vi "Calculate Index Array.vi"(8 "error in (no error)":errorcluster, 10 "3D Surface Datatype.lvclass in":refnum<class "3D Surface Datatype.lvclass">, 11 "Plot Representation In":T1) -> (0 "error out":errorcluster, 2 "3D Surface Datatype.lvclass out":refnum<class "3D Surface Datatype.lvclass">, 3 "Plot Representation Out":T1)   [LabVIEW 2020, in "3D Surface Datatype.lvclass"]
uses:
  <vilib>/Math Plots/3D Math Plots/3D Surface/3D Surface Datatype/3D Surface Datatype.lvclass
  <vilib>/Math Plots/3D Math Plots/3D Plot/3D Plot/Typedef/Plot Representation.ctl
  <vilib>/Math Plots/3D Math Plots/3D Plot/3D Plot/Typedef/Range Clusters.ctl
  <vilib>/Math Plots/3D Math Plots/3D Plot/3D Plot/Typedef/Mesh Data.ctl
  <vilib>/Math Plots/3D Math Plots/3D Plot/3D Plot/3D Plot.lvclass
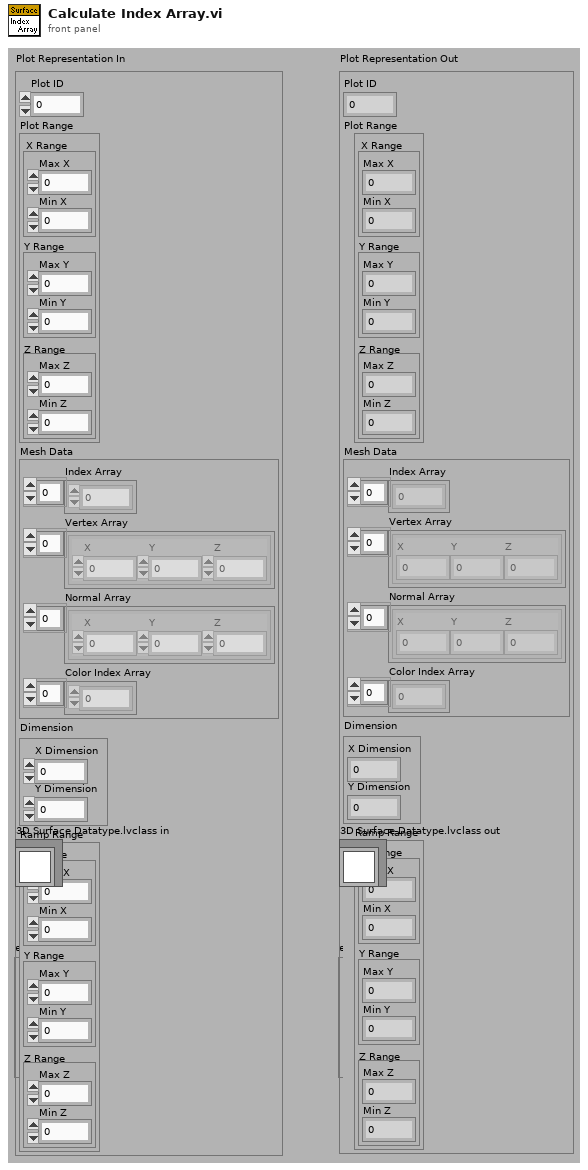
[diagram p1: front panel]
types:
  T1 = typedef "3D Plot.lvclass/Plot Representation.ctl" = cluster{"Plot ID":i32, "Plot Range":T2, "Mesh Data":T3, "Dimension":cluster{"X Dimension":i32, "Y Dimension":i32}, "Ramp Range":T2}
  T2 = typedef "3D Plot.lvclass/Range Clusters.ctl" = cluster{"X Range":cluster{"Max X":sgl, "Min X":sgl}, "Y Range":cluster{"Max Y":sgl, "Min Y":sgl}, "Z Range":cluster{"Max Z":sgl, "Min Z":sgl}}
  T3 = typedef "3D Plot.lvclass/Mesh Data.ctl" = cluster{"Index Array":u32[], "Vertex Array":cluster{"X":sgl, "Y":sgl, "Z":sgl}[], "Normal Array":cluster{"X":sgl, "Y":sgl, "Z":sgl}[], "Color Index Array":i32[]}
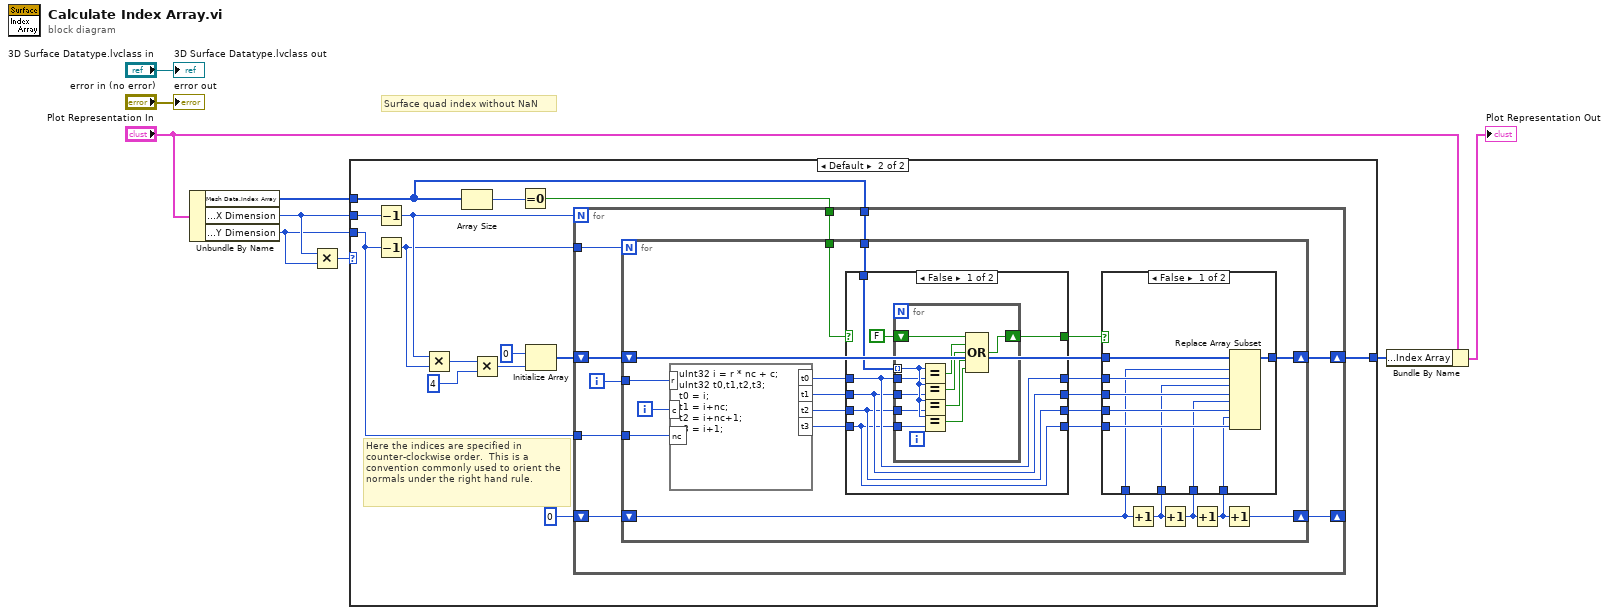
[diagram p0: block diagram]
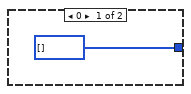
[diagram p2: hidden frame]
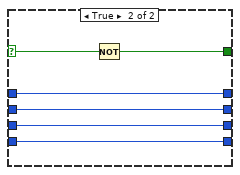
[diagram p3: hidden frame]
diagram:
  # "Surface quad index without NaN"
  n1 = Unbundle By Name("Plot Representation In") -> ("Mesh Data.Index Array"=w1:u32[], "Dimension.X Dimension"=w4:i32, "Dimension.Y Dimension"=w3:i32)
  n2 = Multiply(x=w4, y=w3) -> (x*y=w2:i32)
  n3 = case shown="Default" w2 {
    tunnel: w4 -> [_ w24]
    tunnel: w3 -> [_ w23]
    tunnel: [u32[] [] w22] -> w5
    tunnel: w1 -> [_ w13]
    frame 0 {
    }
    frame Default {
      # "Here the indices are specified in counter-clockwise order.  This is a convention commonly used to orient the normals under the right hand rule."
      n4 = Decrement(x=w24) -> (x-1=w17:i32)
      n5 = Decrement(x=w23) -> (x-1=w16:i32)
      n6 = Multiply(x=w17, y=w16) -> (x*y=w18:i32)
      n7 = Array Size(array=w13) -> (size(s)=w12:i32)
      n8 = Multiply(x=w18, y=4) -> (x*y=w14:i32)
      n9 = Equal To 0?(x=w12) -> (x = 0?=w11:bool)
      n10 = Initialize Array(u32 0, w14) -> (w20:u32[])
      n11 = for {
        N: w17 -> [_]
        shift-right: [w29] -> w22
        shift-left: w20 -> [w33]
        tunnel: w16 -> [w31]
        tunnel: w23 -> [w30]
        shift-right: [w28] -> _
        shift-left: 0 -> [w27]
        tunnel: w13 -> [w26]
        tunnel: w11 -> [w25]
        i -> [w32]
        n12 = for {
          N: w31 -> [_]
          tunnel: w32 -> [w52]
          tunnel: w30 -> [w50]
          shift-right: [w53] -> w29
          shift-left: w33 -> [w54]
          shift-right: [w49] -> w28
          shift-left: w27 -> [w45]
          tunnel: w26 -> [w35]
          tunnel: w25 -> [w42]
          i -> [w51]
          n13 = formula code="uInt32 i = r * nc + c; \nuInt32 t0,t1,t2,t3;\nt0 = i; \nt1 = i+nc; \nt2 = i+nc+1; \nt3 = i+1;"("r"=w52, "nc"=w50, "c"=w51) -> ("t0"=w43:u32, "t1"=w40:u32, "t2"=w38:u32, "t3"=w36:u32)
          n14 = case shown="False" w42 {
            selector: w42 -> [_ w74]
            tunnel: [w58 w78] -> w44
            tunnel: w43 -> [w58 w78]
            tunnel: [w57 w77] -> w41
            tunnel: w40 -> [w57 w77]
            tunnel: [w56 w76] -> w39
            tunnel: w38 -> [w56 w76]
            tunnel: [w55 w75] -> w37
            tunnel: w36 -> [w55 w75]
            tunnel: w35 -> [w61 _]
            tunnel: [w59 w73] -> w34
            frame False {
              n15 = for {
                tunnel: w61 -> [w72] mode=indexing
                tunnel: w58 -> [w71]
                tunnel: w57 -> [w70]
                tunnel: w56 -> [w69]
                tunnel: w55 -> [w68]
                shift-right: [w63] -> w59
                shift-left: FALSE -> [w62]
                n16 = Equal?(x=w72, y=w71) -> (x = y?=w67:bool)
                n17 = Equal?(x=w72, y=w70) -> (x = y?=w66:bool)
                n18 = Equal?(x=w72, y=w69) -> (x = y?=w65:bool)
                n19 = Equal?(x=w72, y=w68) -> (x = y?=w64:bool)
                n20 = Compound Arithmetic op=OR(w62, w67, w66, w65, w64) -> (w63:bool)
              }
            }
            frame True {
              n21 = Not(x=w74) -> (.not. x?=w73:bool)
            }
          }
          n22 = Increment(x=w45) -> (x+1=w46:i32)
          n23 = Increment(x=w46) -> (x+1=w47:i32)
          n24 = Increment(x=w47) -> (x+1=w48:i32)
          n25 = case shown="False" w34 {
            tunnel: w54 -> [w88 w89]
            tunnel: [w87 w89] -> w53
            tunnel: w44 -> [w86 _]
            tunnel: w41 -> [w85 _]
            tunnel: w39 -> [w84 _]
            tunnel: w37 -> [w83 _]
            tunnel: w48 -> [w82 _]
            tunnel: w47 -> [w81 _]
            tunnel: w46 -> [w80 _]
            tunnel: w45 -> [w79 _]
            frame False {
              n26 = Replace Array Subset(array=w88, new element #1=w86, index #1=w79, new element #2=w85, index #2=w80, new element #3=w84, index #3=w81, new element #4=w83, index #4=w82) -> (w87:u32[])
            }
            frame True {
            }
          }
          n27 = Increment(x=w48) -> (x+1=w49:i32)
        }
      }
    }
  }
  n28 = Bundle By Name(cluster="Plot Representation In", "Mesh Data.Index Array"=w5) -> (→"Plot Representation Out":T1)
  "error out" <- "error in (no error)"
  "3D Surface Datatype.lvclass out" <- "3D Surface Datatype.lvclass in"
